vi "Check test 2.vi"(8 "error in (no error)":errorcluster, 10 "Message in":refnum<class "Message.lvclass">, 11 "Test_ExampleClassA in":refnum<class "Test_ExampleClassA.lvclass">) -> (0 "error out":errorcluster, 3 "Test_ExampleClassA out":refnum<class "Test_ExampleClassA.lvclass">)   [LabVIEW 2012, in "Test_ExampleClassA.lvclass"]
doc: "Checks whether subtest 2 was passed (i.e. whether sample production by test subject is properly working)."
uses:
  Test_ExampleClassA.lvclass
  Message/Message.lvclass
  FetchMessage/FetchMessage.lvclass
  TerminateMessage/TerminateMessage.lvclass
  ExampleClassA/Settings cluster.ctl
  Test_ExampleClassA.lvclass/Test_ExampleClassA.ctl
  GenericMessage/GenericMessage.lvclass
  Message/Add or replace parameter.vi
  ExampleClassA/ExampleClassA.lvclass
  Murmex/Murmex.lvclass
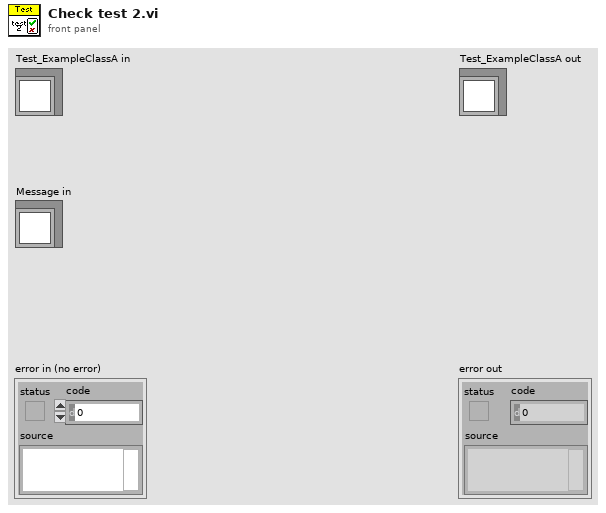
[diagram p1: front panel]
types:
  T1 = typedef "ExampleClassA.lvclass/Settings cluster.ctl" = cluster{"period?":dbl[unit], "number of blocks":i32, "number of channels":i32}
  T2 = typedef "Murmex.lvlib/Murmex.lvclass/command_enum.ctl" = enum16{"null", "initialise", "reset", "terminate", "acknowledge", "update", "inspect", "inform", "proceed", "start", "stop", "fetch", "configure", "generic"}
  T3 = typedef "Murmex.lvlib/FetchMessage.lvclass/Channel data cluster.ctl" = cluster{"channel id":i32, "data UInt8":u8[], "data type":T4, "dimensions":i32[], "physical units":T5[], "waveform dt":dbl, "waveform":T6}
  T4 = typedef "Murmex.lvlib/Murmex.lvclass/data_type_enum.ctl" = enum16{"Float128", "Float64", "Float32", "Int64", "Int32", "Int16", "Int8", "UInt64", "UInt32", "UInt16", "UInt8", "Boolean", "String"}
  T5 = typedef "Physical Units__ogtk.ctl" = cluster{"Base Units":enum16{"radian", "steradian", "second", "meter", "kilogram", "ampere", "kelvin", "mole", "candela"}, "Exponent":i16}
  T6 = typedef "Murmex.lvlib/Murmex.lvclass/waveform_type_enum.ctl" = enum16{"no waveform", "analog", "digital"}
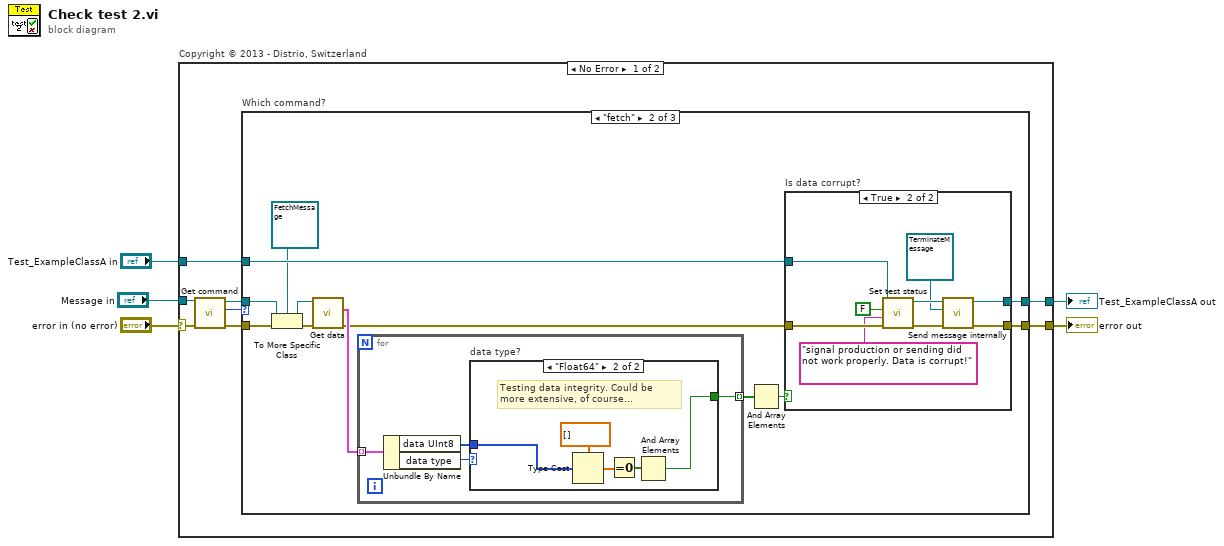
[diagram p0: block diagram]
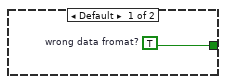
[diagram p3: hidden frame]
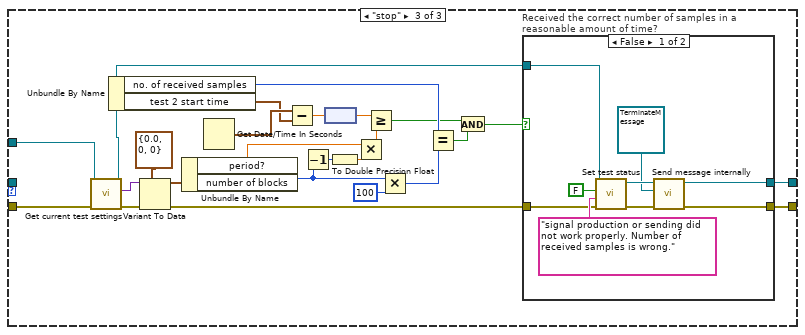
[diagram p5: hidden frame]
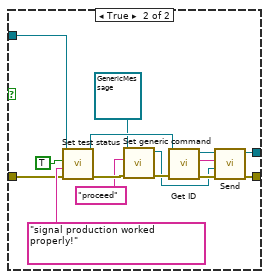
[diagram p6: hidden frame]
diagram:
  n1 = case "Copyright © 2013 - Distrio, Switzerland" shown="No Error" "error in (no error)" {
    selector: "error in (no error)" -> [w9 w99]
    tunnel: [w12 w99] -> w4
    tunnel: [w11 w98] -> w2
    tunnel: "Test_ExampleClassA in" -> [w13 w98]
    tunnel: "Message in" -> [w10 _]
    frame No Error {
      n2 = call "Get command.vi"("error in (no error)"=w9, "Message in"=w10) -> ("error out"=w8:errorcluster, "command"=w7:T2, "Message out"=w6:refnum<class "Message.lvclass">)  [unwired: 7 in]
      n3 = case "Which command?" shown="\"fetch\"" w7 {
        tunnel: w13 -> [w15 w24 w69]
        tunnel: [w14 w25 w65] -> w12
        tunnel: [w15 w23 w63] -> w11
        tunnel: w8 -> [w14 w20 w49]
        tunnel: w6 -> [_ w22 _]
        frame Default {
        }
        frame "fetch" {
          n4 = To More Specific Class(target class=refnum<class "FetchMessage.lvclass"> refnum ("FetchMessage.lvclass"), reference=w22, error in=w20) -> (specific class reference=w21:refnum<class "FetchMessage.lvclass">, error out=w19:errorcluster)
          n5 = call "Get data.vi"("error in (no error)"=w19, "FetchMessage.lvclass"=w21) -> ("error out"=w26:errorcluster, "data (channels)"=w27:T3[])  [unwired: 7 in, 1 out]
          n6 = for {
            tunnel: w27 -> [w30] mode=indexing
            tunnel: [w31] -> w16 mode=indexing
            n7 = Unbundle By Name(w30) -> ("data UInt8"=w28:u8[], "data type"=w29:T4)
            n8 = case "data type?" shown="\"Float64\"" w29 {
              tunnel: [w32 w34] -> w31
              tunnel: w28 -> [_ w33]
              frame Default {
                w32 = TRUE  # wrong data fromat?
              }
              frame "Float64" {
                # "Testing data integrity. Could be more extensive, of course..."
                n9 = Type Cast(type=dbl[] [] ("data (UInt8)"), x=w33) -> (*(type *) &x=w36:dbl[])
                n10 = Equal To 0?(x=w36) -> (x = 0?=w35:bool[])
                n11 = And Array Elements(Boolean array=w35) -> (logical AND=w34:bool)
              }
            }
          }
          n12 = And Array Elements(Boolean array=w16) -> (logical AND=w17:bool)
          n13 = case "Is data corrupt?" shown="True" w17 {
            tunnel: w26 -> [w39 w47]
            tunnel: w24 -> [w38 w46]
            tunnel: [w39 w43] -> w25
            tunnel: [w38 w42] -> w23
            frame False {
            }
            frame True {
              n14 = call-dynamic "Set test status.vi"("error in (no error)"=w47, "details"="signal production or sending did not work properly. Data is corrupt!", "passed?"=FALSE, "MurmexTest in"=w46) -> ("error out"=w44:errorcluster, "MurmexTest out"=w41:refnum<class "Test_ExampleClassA.lvclass">)  [unwired: 6 in]
              n15 = call "Send message internally.vi"("error in (no error)"=w44, "Message"=refnum<class "TerminateMessage.lvclass"> refnum ("TerminateMessage.lvclass"), "Murmex in"=w41) -> ("error out"=w43:errorcluster, "Murmex out"=w42:refnum<class "Test_ExampleClassA.lvclass">)  [unwired: 7 in]
            }
          }
        }
        frame "stop" {
          n16 = call-dynamic "Get current test settings.vi"("error in (no error)"=w49, "MurmexTest in"=w69) -> ("error out"=w73:errorcluster, "settings"=w72:variant, "MurmexTest out"=w64:refnum<class "Test_ExampleClassA.lvclass">)  [unwired: 4 in, 3 out]
          n17 = Unbundle By Name(w64) -> ("no. of received samples"=w67:i32, "test 2 start time"=w61:timestamp)
          n18 = Variant To Data(error in=w73, type=T1 {"period?"=0.0, "number of blocks"=0, "number of channels"=0} ("settings"), Variant=w72) -> (data=w70:T1, error out=w66:errorcluster)
          n19 = Unbundle By Name(w70) -> ("period?"=w60:dbl[unit], "number of blocks"=w57:i32)
          n20 = Get Date/Time In Seconds() -> (seconds since 1Jan1904=w62:timestamp)
          n21 = Subtract(x=w62, y=w61) -> (x-y=w54:dbl)
          n22 = Decrement(x=w57) -> (x-1=w59:i32)
          n23 = node(w54) -> (w53:dbl[unit])
          n24 = To Double Precision Float(number=w59) -> (double precision float=w58:dbl)
          n25 = Multiply(x=w60, y=w58) -> (x*y=w55:dbl[unit])
          n26 = Greater Or Equal?(x=w53, y=w55) -> (x >= y?=w52:bool)
          n27 = Multiply(x=w57, y=100 ("x")) -> (x*y=w68:i32)
          n28 = Equal?(x=w67, y=w68) -> (x = y?=w51:bool)
          n29 = And(x=w52, y=w51) -> (x .and. y?=w50:bool)
          n30 = case "Received the correct number of samples in a reasonable amount of time?" shown="False" w50 {
            tunnel: w66 -> [w80 w95]
            tunnel: [w77 w92] -> w65
            tunnel: w64 -> [w79 w94]
            tunnel: [w76 w91] -> w63
            frame False {
              n31 = call-dynamic "Set test status.vi"("error in (no error)"=w80, "details"="signal production or sending did not work properly. Number of received samples is wrong.", "passed?"=FALSE, "MurmexTest in"=w79) -> ("error out"=w74:errorcluster, "MurmexTest out"=w78:refnum<class "Test_ExampleClassA.lvclass">)  [unwired: 6 in]
              n32 = call "Send message internally.vi"("error in (no error)"=w74, "Message"=refnum<class "TerminateMessage.lvclass"> refnum ("TerminateMessage.lvclass"), "Murmex in"=w78) -> ("error out"=w77:errorcluster, "Murmex out"=w76:refnum<class "Test_ExampleClassA.lvclass">)  [unwired: 7 in]
            }
            frame True {
              n33 = call-dynamic "Set test status.vi"("error in (no error)"=w95, "details"="signal production worked properly!", "passed?"=TRUE, "MurmexTest in"=w94) -> ("error out"=w87:errorcluster, "MurmexTest out"=w93:refnum<class "Test_ExampleClassA.lvclass">)  [unwired: 6 in]
              n34 = call "Set generic command.vi"("error in (no error)"=w87, "generic command"="proceed", "GenericMessage in"=refnum<class "GenericMessage.lvclass"> refnum ("GenericMessage.lvclass")) -> ("error out"=w86:errorcluster, "GenericMessage out"=w83:refnum<class "GenericMessage.lvclass">)  [unwired: 7 in]
              n35 = call "Get ID.vi"("error in (no error)"=w86, "Murmex in"=w93) -> ("error out"=w88:errorcluster, "component id"=w89:string, "Murmex out"=w90:refnum<class "Test_ExampleClassA.lvclass">)  [unwired: 7 in]
              n36 = call "Send.vi"("error in (no error)"=w88, "Message"=w83, "recipient"=w89, "Murmex in"=w90) -> ("error out"=w92:errorcluster, "Murmex out"=w91:refnum<class "Test_ExampleClassA.lvclass">)  [unwired: 6 in]
            }
          }
        }
      }
    }
    frame Error {
    }
  }
  "error out" <- w4
  "Test_ExampleClassA out" <- w2
